vi "求平均数while.vi"(1 "B":dbl, 2 "A":dbl) -> (0 "Result":dbl)   [LabVIEW 2017]
panel:
  in  "?":bool
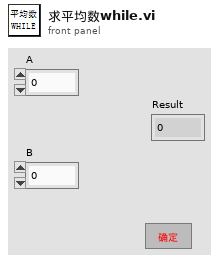
[diagram p1: front panel]
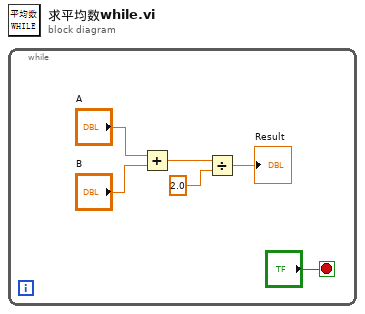
[diagram p0: block diagram]
diagram:
  n1 = while {
    stop <- "?" stop-if-true
    n2 = Add(x="A", y="B") -> (x+y=w4:dbl)
    n3 = Divide(x=w4, y=2.0) -> (x/y=→"Result":dbl)
  }
